vi "ReferenceScanViParameters.vi"(8 "error in":errorcluster) -> (0 "error out":errorcluster, 2 "Labels":string[](array[string]), 3 "ScanParameters[]":refnum<vi>[](array[refnum]))   [LabVIEW 2016]
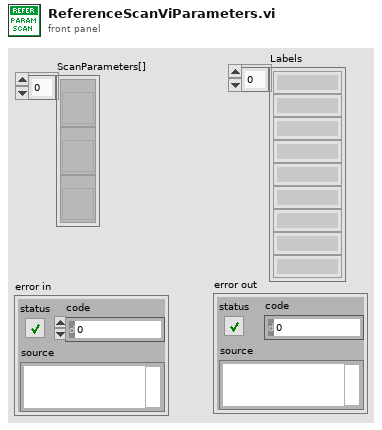
[diagram p1: front panel]
types:
  T1 = enum32{"Bad", "Idle", "Run top level", "Running"}
  T2 = enum32{"Invalid", "Standard", "Closed", "Hidden", "Minimized", "Maximized"}
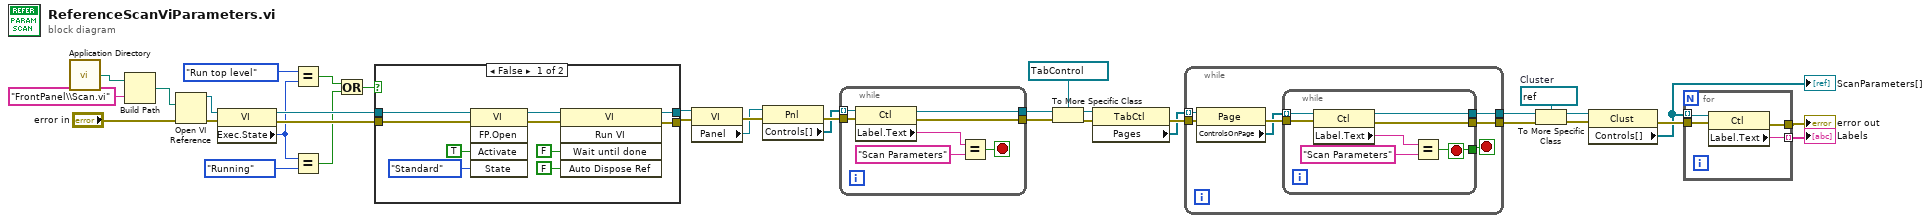
[diagram p0: block diagram]
diagram:
  w16 = refnum<vi> refnum  # Cluster
  n1 = call <vilib>:"Application Directory.vi"() -> ("Application Directory"=w30:path)
  n2 = Build Path(base path=w30, name or relative path="FrontPanel\\Scan.vi") -> (appended path=w29:path)
  n3 = Open VI Reference(vi path=w29, error in (no error)="error in") -> (vi reference=w1:refnum<vi>, error out=w2:errorcluster)  [unwired: 4 in]
  n4 = property class="VI"(reference=w1, error in=w2) -> (reference out=w12:refnum<vi>, error out=w11:errorcluster, "Exec.State"=w6:T1)
  n5 = Equal?(x=T1."Run top level" ("Execution:State"), y=w6) -> (x = y?=w8:bool)
  n6 = Equal?(x=w6, y=T1."Running" ("Execution:State")) -> (x = y?=w7:bool)
  n7 = Or(x=w8, y=w7) -> (x .or. y?=w5:bool)
  n8 = case shown="False" w5 {
    tunnel: [w41 w47] -> w4
    tunnel: [w40 w48] -> w3
    tunnel: w12 -> [w38 w48]
    tunnel: w11 -> [w37 w47]
    frame False {
      n9 = invoke class="VI" method="FP.Open"(reference=w38, error in=w37, "Activate"=TRUE ("Activate?"), "State"=T2."Standard") -> (reference out=w43:refnum<vi>, error out=w42:errorcluster)  [unwired: 1 in, 3 out]
      n10 = invoke class="VI" method="Run VI"(reference=w43, error in=w42, "Wait until done"=FALSE ("Wait Until Done"), "Auto Dispose Ref"=FALSE ("Auto Dispose Reference")) -> (reference out=w40:refnum<vi>, error out=w41:errorcluster)  [unwired: 1 in, 3 out]
    }
    frame True {
    }
  }
  n11 = property class="VI"(reference=w3, error in=w4) -> (error out=w35:errorcluster, "Panel"=w28:refnum<vi>)  [unwired: 1 out]
  n12 = property class="Pnl"(reference=w28, error in=w35) -> (error out=w36:errorcluster, "Controls[]"=w32:refnum<vi>[])  [unwired: 1 out]
  n13 = while {
    tunnel: w32 -> [w55] mode=indexing
    tunnel: [w53] -> w33
    tunnel: [w52] -> w34
    tunnel: w36 -> [w51]
    stop <- w49 stop-if-true
    n14 = property class="Ctl"(reference=w55, error in=w51) -> (reference out=w53:refnum<vi>, error out=w52:errorcluster, "Label.Text"=w50:string)
    n15 = Equal?(x=w50, y="Scan Parameters") -> (x = y?=w49:bool)
  }
  n16 = To More Specific Class(target class=refnum<vi> refnum ("Menus"), reference=w33, error in=w34) -> (specific class reference=w21:refnum<vi>, error out=w26:errorcluster)
  n17 = property class="TabCtl"(reference=w21, error in=w26) -> (error out=w25:errorcluster, "Pages"=w22:refnum<vi>[])  [unwired: 1 out]
  n18 = while {
    tunnel: w22 -> [w61] mode=indexing
    tunnel: [w58] -> w23
    tunnel: [w57] -> w24
    tunnel: w25 -> [w56]
    stop <- w59 stop-if-true
    n19 = property class="Page"(reference=w61, error in=w56) -> (error out=w62:errorcluster, "ControlsOnPage"=w60:refnum<vi>[])  [unwired: 1 out]
    n20 = while {
      tunnel: w60 -> [w69] mode=indexing
      tunnel: [w67] -> w59
      tunnel: [w66] -> w58
      tunnel: [w65] -> w57
      tunnel: w62 -> [w64]
      stop <- w67 stop-if-true
      n21 = property class="Ctl"(reference=w69, error in=w64) -> (reference out=w66:refnum<vi>, error out=w65:errorcluster, "Label.Text"=w63:string)
      n22 = Equal?(x=w63, y="Scan Parameters") -> (x = y?=w67:bool)
    }
  }
  n23 = To More Specific Class(target class=w16, reference=w23, error in=w24) -> (specific class reference=w17:refnum<vi>, error out=w18:errorcluster)
  n24 = property class="Clust"(reference=w17, error in=w18) -> (error out=w19:errorcluster, "Controls[]"=w13:refnum<vi>[])  [unwired: 1 out]
  "ScanParameters[]" <- w13
  n25 = for {
    tunnel: w13 -> [w73] mode=indexing
    tunnel: w19 -> [w72]
    tunnel: [w71] -> w14
    tunnel: [w70] -> w15 mode=indexing
    n26 = property class="Ctl"(reference=w73, error in=w72) -> (error out=w71:errorcluster, "Label.Text"=w70:string)  [unwired: 1 out]
  }
  "Labels" <- w15
  "error out" <- w14
